vi "U6 eAIN with Loop and Chart.vi"() -> (0 "error out":errorcluster)   [LabVIEW 2021]
panel:
  in  "Interval (ms)":u32=500
  in  "stop":bool
  out "Waveform Chart":dbl(graph)
  in  "FirstFound":bool=TRUE
  in  "Address":string="1"
  in  "ChannelP":i32
  out "Error Message":string="No Error"
  out "Value Read":dbl format="%.6f"
  # "Reads 1 analog input using the UD easy function eAIN."
  # "14 = Temp degC\n15 = GND"
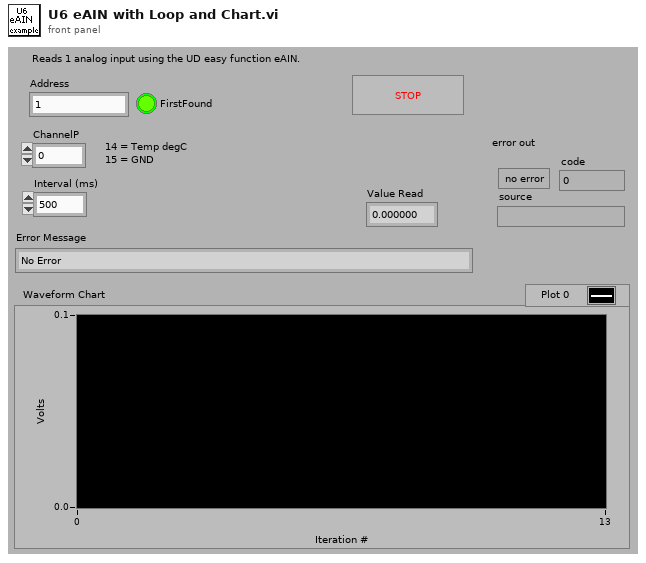
[diagram p1: front panel]
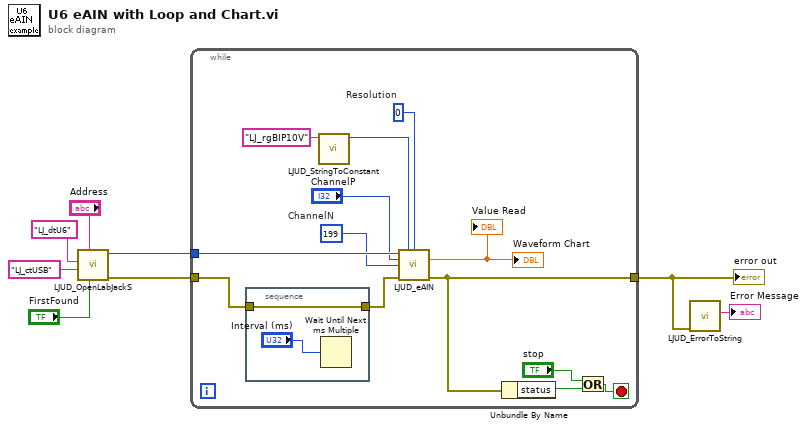
[diagram p0: block diagram]
diagram:
  n1 = call "LJUD_OpenLabJackS.vi"("FirstFound"="FirstFound", "Address"="Address", "ConnectionType"="LJ_ctUSB", "DeviceType"="LJ_dtU6") -> ("error out"=w1:errorcluster, "Handle"=w4:i32)  [unwired: 5 in, 1 out]
  n2 = while {
    tunnel: w1 -> [w10]
    tunnel: w4 -> [w21]
    tunnel: [w12] -> w7
    stop <- w14 stop-if-true
    w16 = 0  # Resolution
    w17 = 199  # ChannelN
    n3 = stacked-sequence {
      tunnel: w10 -> [w23]
      tunnel: [w23] -> w9
      frame #0 {
        n4 = Wait Until Next ms Multiple(millisecond multiple="Interval (ms)") -> ()  [unwired: 1 out]
      }
    }
    n5 = call "LJUD_StringToConstant.vi"("String"="LJ_rgBIP10V") -> ("Constant Number"=w20:i32)  [unwired: 9 in, 1 out]
    n6 = call "LJUD_eAIN.vi"("Handle In"=w21, "Range"=w20, "Resolution"=w16, "ChannelP"="ChannelP", "ChannelN"=w17, "error in"=w9) -> ("Voltage"=→"Value Read" →"Waveform Chart":dbl, "error out"=w12:errorcluster)  [unwired: 7 in, 1 out]
    n7 = Unbundle By Name(w12) -> ("status"=w13:bool)
    n8 = Or(x="stop", y=w13) -> (x .or. y?=w14:bool)
  }
  "error out" <- w7
  n9 = call "LJUD_ErrorToString.vi"("error in"=w7) -> ("String"=→"Error Message":string)  [unwired: 10 in]
